vi "MB MFC Flow.vi"(8 "error in (no error)":errorcluster, 11 "TCP Ref":refnum<k5>) -> (0 "error out":errorcluster, 1 "Flow(sccm)":sgl, 3 "dup TCP Ref":refnum<k5>)   [LabVIEW 2011]
doc: "This VI reads the flow from an MKS Modbus MFC."
uses:
  EtherNet.lib/Modbus/mb Ethernet.llb/MB Modbus Command.ctl
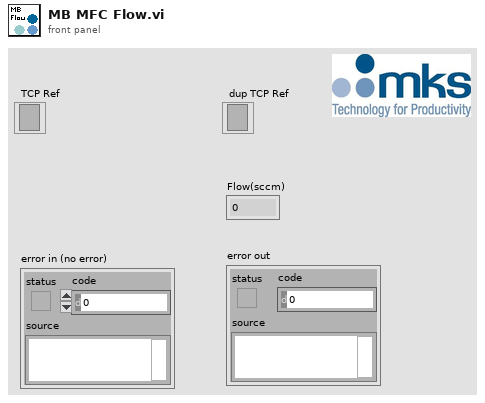
[diagram p1: front panel]
types:
  T1 = typedef "MB Modbus Command.ctl" = cluster{"Function Code":u8, "Starting Address":u16, "Quantity":u16, "Data":u16[], "Discrete":bool[]}
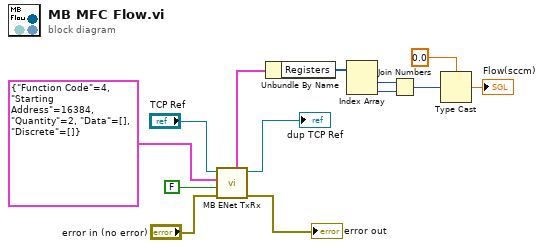
[diagram p0: block diagram]
diagram:
  n1 = call "MB ENet TxRx.vi"("error in (no error)"="error in (no error)", "Use MODBUS Data Unit?"=FALSE, "Modbus Command"=T1 {"Function Code"=4, "Starting Address"=16384, "Quantity"=2, "Data"=[], "Discrete"=[]}, "TCP Ref:ValBlock"="TCP Ref") -> ("error out"=→"error out":errorcluster, "dup TCP Ref:ValBlock"=→"dup TCP Ref":refnum<k5>, "Registers"=w11:cluster{"Registers":u16[], "Discrete":bool[]})  [unwired: 3 in, 2 out]
  n2 = Unbundle By Name(w11) -> ("Registers"=w10:u16[])
  n3 = Index Array(array=w10) -> (element #1=w9:u16, element #2=w8:u16)  [unwired: 2 in]
  n4 = Join Numbers(hi=w9, lo=w8) -> ((hi.lo)=w7:u32)
  n5 = Type Cast(type=sgl 0.0 ("element"), x=w7) -> (*(type *) &x=→"Flow(sccm)":sgl)
